vi "Set Data in Group Buffer.vi"(9 "New Trigger":bool, 10 "Data in":dbl[](array[numeric]), 11 "Group Buffer Data in":T1) -> (1 "Buffer Full":bool, 2 "Flush Pretrigger Data":bool, 3 "Group Buffer Data out":T1)   [LabVIEW 2027, in "Embedded Data Logger Engine.lvlib"]
uses:
  Embedded Data Logger Engine.lvlib
  Group Buffer Data.ctl
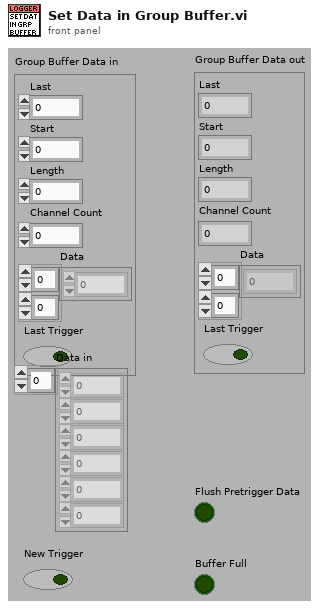
[diagram p1: front panel]
types:
  T1 = typedef "Embedded Data Logger Engine.lvlib/Group Buffer Data.ctl" = cluster{"Last":i32, "Start":i32, "Length":i32, "Channel Count":i32, "Data":dbl[][], "Last Trigger":bool}
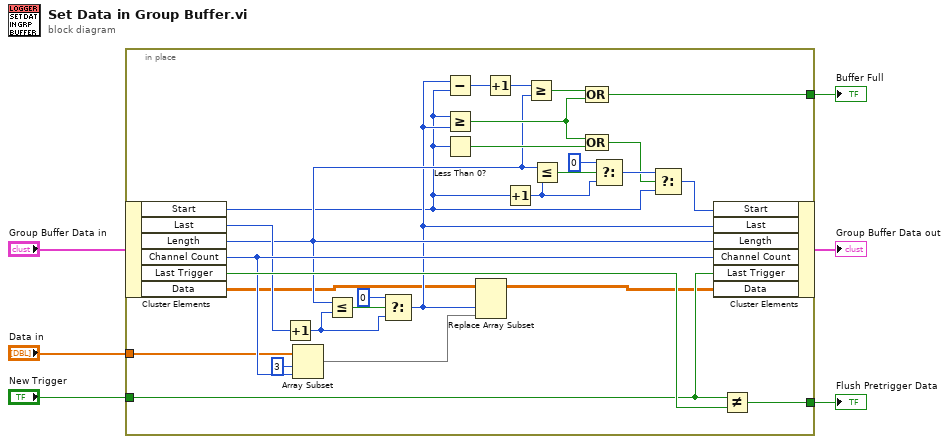
[diagram p0: block diagram]
diagram:
  n1 = in-place {
    in-place-border: "Data in" -> [w27]
    in-place-border: [w20] -> w3
    in-place-border: "New Trigger" -> [w17]
    in-place-border: [w16] -> w1
    n2 = in-place-cluster #1("Group Buffer Data in") -> ("Start"=w8:i32, "Last"=w19:i32, "Length"=w18:i32, "Channel Count"=w28:i32, "Last Trigger"=w34:bool, "Data"=w14:dbl[][])
    n3 = Increment(x=w19) -> (x+1=w29:i32)
    n4 = Array Subset(array=w27, index=3, length=w28) -> (w32:dbl[])
    n5 = Less Or Equal?(x=w18, y=w29) -> (x <= y?=w31:bool)
    n6 = Select(t=0 ("f"), s=w31, f=w29) -> (s? t:f=w15:i32)
    n7 = Subtract(x=w15, y=w8) -> (x-y=w24:i32)
    n8 = Greater Or Equal?(x=w8, y=w15) -> (x >= y?=w21:bool)
    n9 = Less Than 0?(x=w8) -> (x < 0?=w25:bool)
    n10 = Replace Array Subset(array=w14, new element=w32, index (col)=w15) -> (w13:dbl[][])  [unwired: 1 in]
    n11 = Increment(x=w24) -> (x+1=w23:i32)
    n12 = Increment(x=w8) -> (x+1=w12:i32)
    n13 = Greater Or Equal?(x=w23, y=w18) -> (x >= y?=w22:bool)
    n14 = Less Or Equal?(x=w18, y=w12) -> (x <= y?=w10:bool)
    n15 = Compound Arithmetic op=OR(w22, w21) -> (w20:bool)
    n16 = Compound Arithmetic op=OR(w21, w25) -> (w9:bool)
    n17 = Select(t=0 ("f"), s=w10, f=w12) -> (s? t:f=w33:i32)
    n18 = Select(t=w33, s=w9, f=w8) -> (s? t:f=w7:i32)
    n19 = in-place-cluster #1("Start"=w7, "Last"=w15, "Length"=w18, "Channel Count"=w28, "Last Trigger"=w17, "Data"=w13) -> (→"Group Buffer Data out":T1)
    n20 = Not Equal?(x=w17, y=w34) -> (x != y?=w16:bool)
  }
  "Buffer Full" <- w3
  "Flush Pretrigger Data" <- w1
